vi "Configure FFT Measurement Control.vi"(6 "Measurement Detector (Peak)":i32(ring) items=["Peak", "RMS"], 7 "FFT Length (2048)":i32=2048, 8 "error in (no error)":errorcluster, 9 "Frequency Span (10MHz)":dbl=10000000.0 format="%#.9p", 10 "Instance (1)":i32=1, 11 "VISA resource name":refnum<visa-resource-name>) -> (0 "error out":errorcluster, 3 "VISA resource name out":refnum<visa-resource-name>)   [LabVIEW 2015, in "Rohde&Schwarz CMXP GPRF.lvlib"]
doc: "Configures FFT Spectrum Analyzer measurement control parameters\n\nAttributes:\nRSCMXPGPRF_ATTR_FFT_MEASUREMENT_FREQUENCY_SPAN\nRSCMXPGPRF_ATTR_FFT_MEASUREMENT_FFT_LENGTH\nRSCMXPGPRF_ATTR_FFT_MEASUREMENT_DETECTOR\n\nRemote-control commands:\nCONFigure:GPRF:MEAS<i>:FFTSanalyzer:FSPan\nCONFigure:GPRF:MEAS<i>:FFTSanalyzer:FFTLength\nCONFigure:GPRF:MEAS<i>:FFTSanalyzer:DETector"
uses:
  <instrlib>/Rohde&Schwarz CMXP GPRF/Rohde&Schwarz CMXP GPRF.lvlib
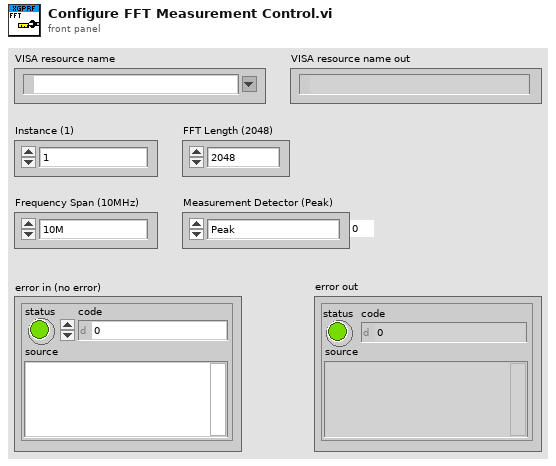
[diagram p1: front panel]
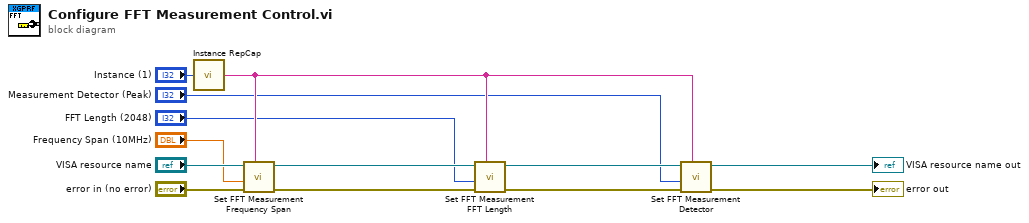
[diagram p0: block diagram]
diagram:
  n1 = call <instrlib>:"Instance RepCap.vi"("instance  in"="Instance (1)") -> ("instance out"=w8:string)
  n2 = call "Set FFT Measurement Frequency Span"("Repeated Capabilities"=w8, "error in (no error)"="error in (no error)", "FFT Measurement Frequency Span (0.0)"="Frequency Span (10MHz)", "instrument handle"="VISA resource name") -> ("error out"=w9:errorcluster, "instrument handle out"=w10:refnum<visa-resource-name>)  [unwired: 6 in]
  n3 = call "Set FFT Measurement FFT Length"("Repeated Capabilities"=w8, "error in (no error)"=w9, "FFT Measurement FFT Length (0)"="FFT Length (2048)", "instrument handle"=w10) -> ("error out"=w5:errorcluster, "instrument handle out"=w4:refnum<visa-resource-name>)  [unwired: 6 in]
  n4 = call "Set FFT Measurement Detector"("Repeated Capabilities"=w8, "error in (no error)"=w5, "FFT Measurement Detector (0 - Peak)"="Measurement Detector (Peak)", "instrument handle"=w4) -> ("error out"=→"error out":errorcluster, "instrument handle out"=→"VISA resource name out":refnum<visa-resource-name>)  [unwired: 6 in]
